vi "Meas_EIS_Spectra_Polar_v6.vi"(9 "output cluster":T1, 10 "testp":T2={"Start F"=1.0, "Stop F"=10000.0, "# Steps"=50, "Init Z Guess"=1.0, "Device #"=0, "Vdrive (V)"=0.1} caption="Test Parameters" {"Vdrive (V)" min=0.0001 max=10; "Device #" min=0 max=10 step=1; "Init Z Guess" format="%_5f"; "# Steps" min=1 max=1800 step=1; "Stop F" min=0.0010000000474974513 max=2000000.0 step=0.001 format="%#_3f"; "Start F" min=0.0010000000474974513 max=2000000.0 step=0.001 format="%#_3f"}, 11 "Output file refnum":refnum<file>) -> ()   [LabVIEW 2018]
uses:
  AC States cntrl.ctl
panel:
  out "Init Z Guess":sgl
  in  "Tab Control":enum32{"Outputs", "TakeData"}(tab)
  out "XY Graph":cluster{sgl, sgl}[](graph)
  out "IERange":i32
  out "IchRange":i32
  out "VchRange":i32
  out "Index no.":i32=1
  out "Zphz":dbl
  out "Zmod":dbl
  out "Zfreq":dbl
  in  "Control Mode":i32(ring)=1 items=["GstatMode", "PstatMode", "ZRAMode", "FRAMode"]
  out "Data Available":bool
  out "Status":enum16{"Ok", "Retry", "Error", "Done"}(ring)
  out "NumPoints":i32
  in  "Freqin":sgl=1000.0 format="%#_3g"
  out "event callback refnum":refnum<k27>
  out "Section":string
  out "ReadZ":refnum<k7>
  out "Pstat":refnum<k7>
  out "Device List":refnum<k7>
  out "Data Acquisition Complete":bool
  in  "GAMRYCOMLib.IGamryReadZ":refnum<k7>
  in  "GAMRYCOMLib.IGamryPstat":refnum<k7>
  in  "GAMRYCOMLib.IGamryDeviceList":refnum<k7>
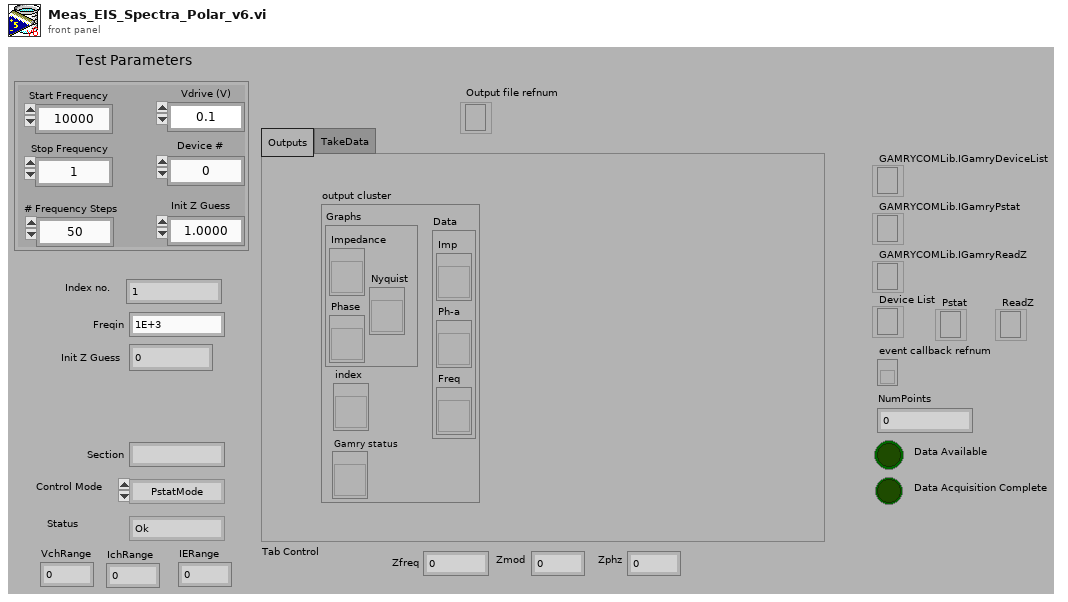
[diagram p1: front panel]
types:
  T1 = cluster{"Data":cluster{"Imp":refnum<vi>, "Ph-a":refnum<vi>, "Freq":refnum<vi>}, "Graphs":cluster{"Impedance":refnum<vi>, "Phase":refnum<vi>, "Nyquist":refnum<vi>}, "index":refnum<vi>, "Gamry status":refnum<vi>}
  T2 = cluster{"Start F":dbl, "Stop F":dbl, "# Steps":u32, "Init Z Guess":sgl, "Device #":i16, "Vdrive (V)":sgl}
  T3 = typedef "AC States cntrl.ctl" = enum16{"Initialize Variables", "Initialize Pstat", "Initialize Dtaq", "Settings", "Frequency calc", "Set Cycle Limits", "Take Data", "Read Z Measure", "Cleanup", "Stop"}
  T4 = cluster{"Imp":refnum<vi>, "Ph-a":refnum<vi>, "Freq":refnum<vi>}
  T5 = cluster{"Impedance":refnum<vi>, "Phase":refnum<vi>, "Nyquist":refnum<vi>}
  T6 = cluster{"Data Acquisition Complete":refnum<vi>, "Status":refnum<vi>}
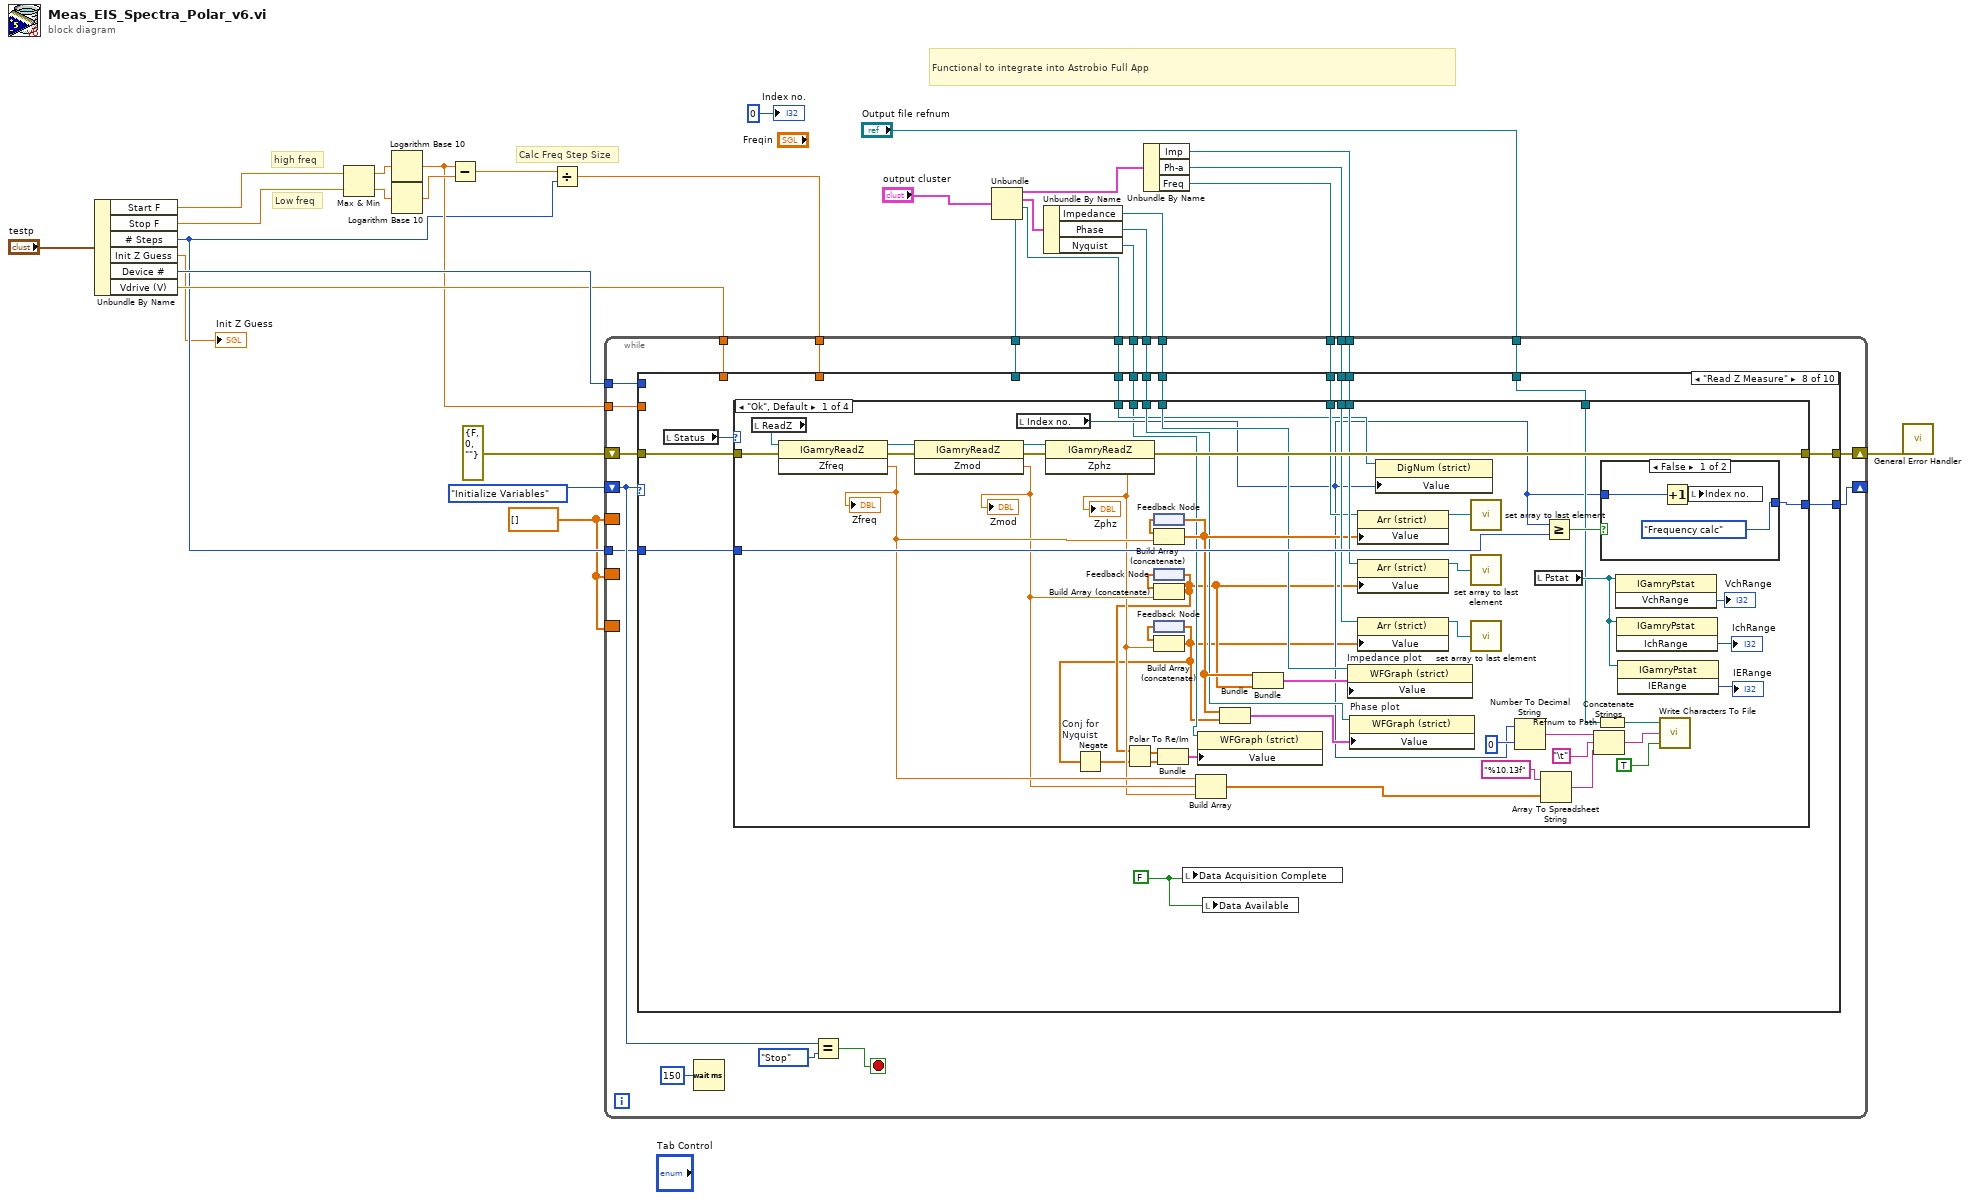
[diagram p0: block diagram]
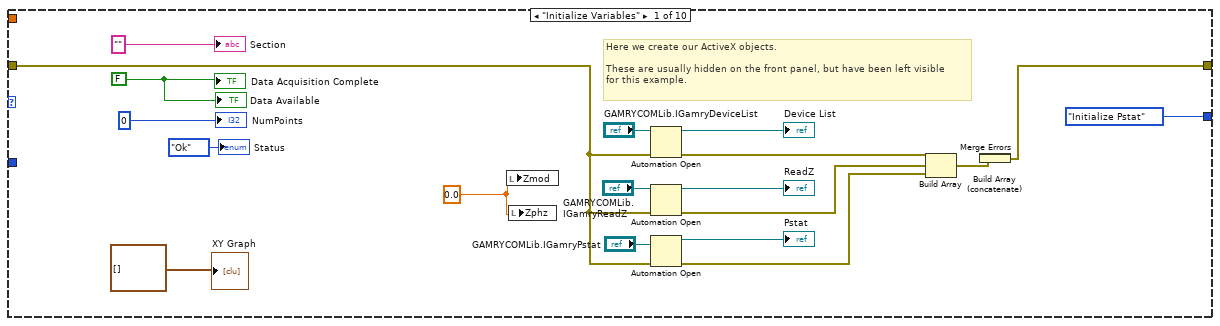
[diagram p2: hidden frame]
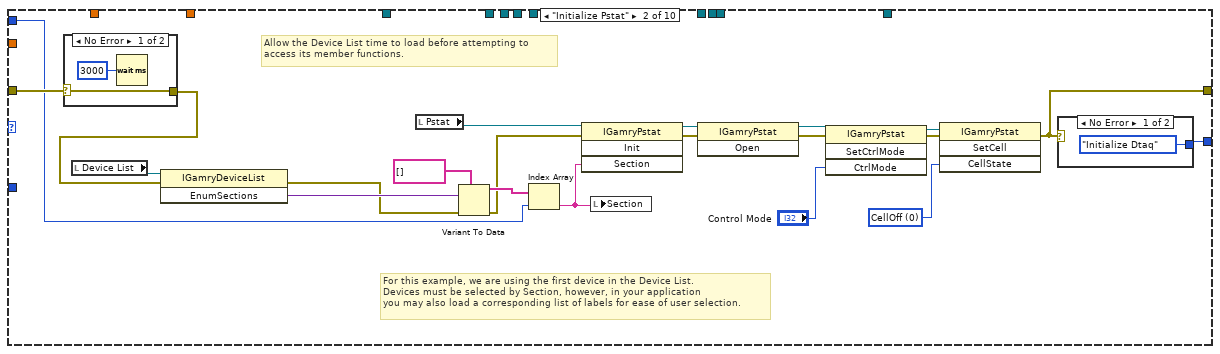
[diagram p3: hidden frame]
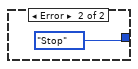
[diagram p5: hidden frame]
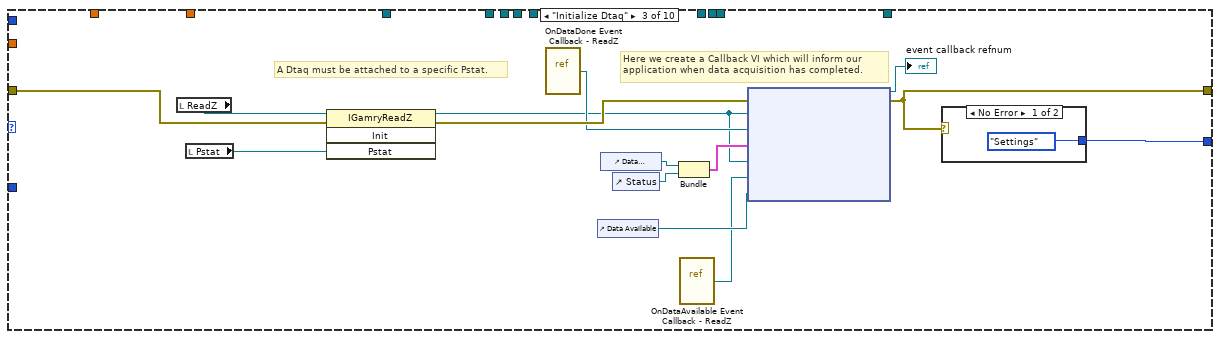
[diagram p6: hidden frame]
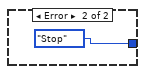
[diagram p7: hidden frame]
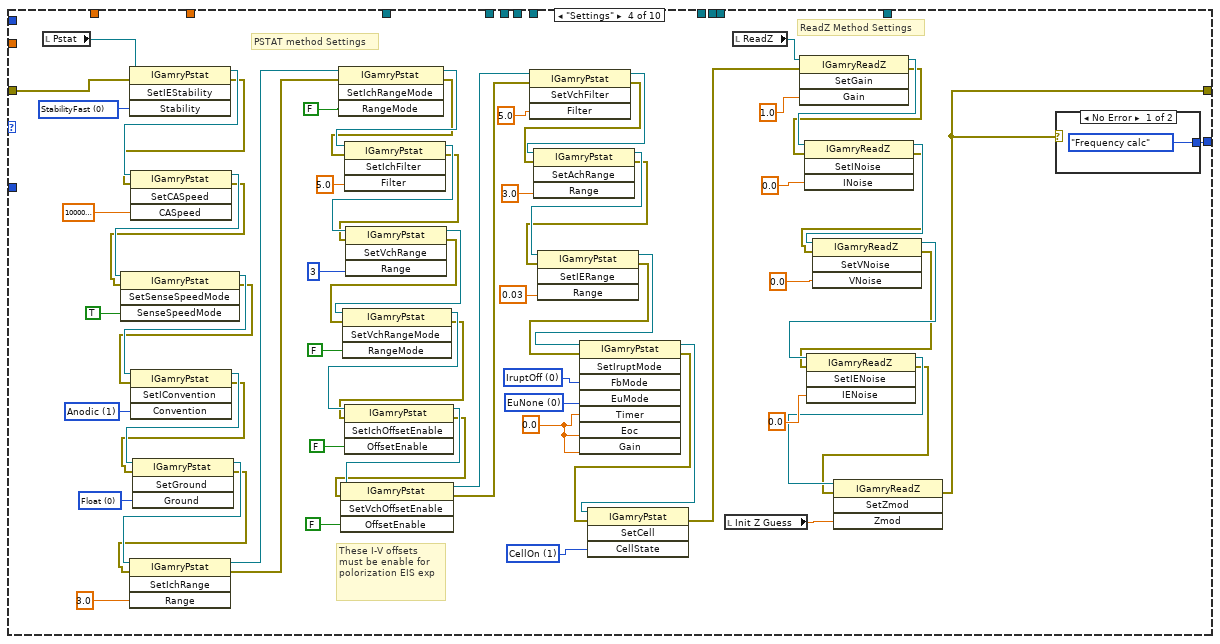
[diagram p8: hidden frame]
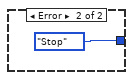
[diagram p9: hidden frame]
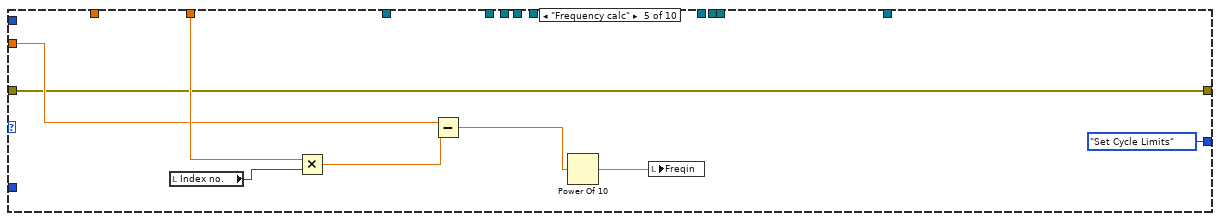
[diagram p10: hidden frame]
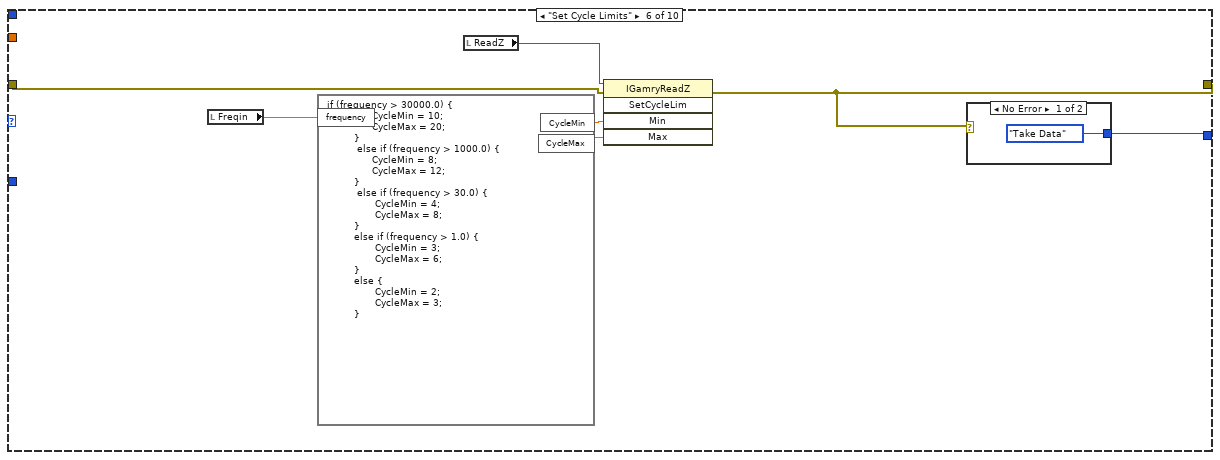
[diagram p11: hidden frame]
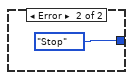
[diagram p12: hidden frame]
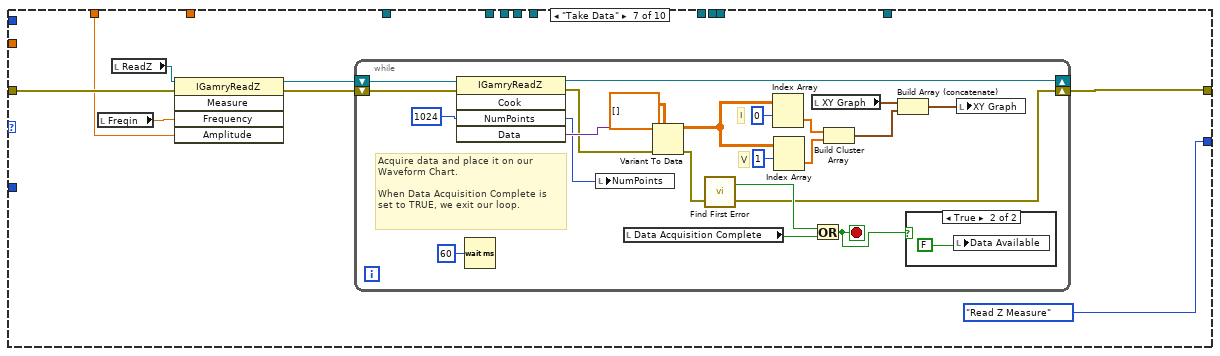
[diagram p13: hidden frame]
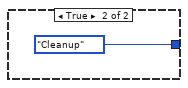
[diagram p15: hidden frame]
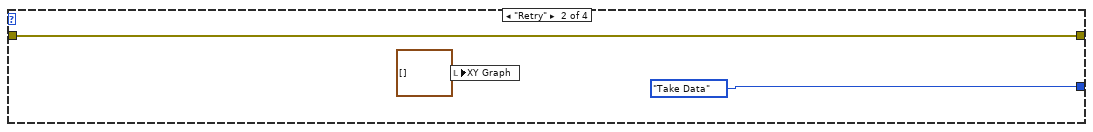
[diagram p16: hidden frame]
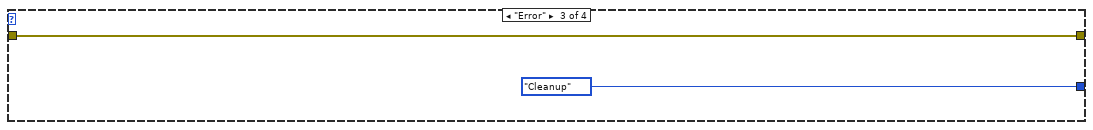
[diagram p17: hidden frame]
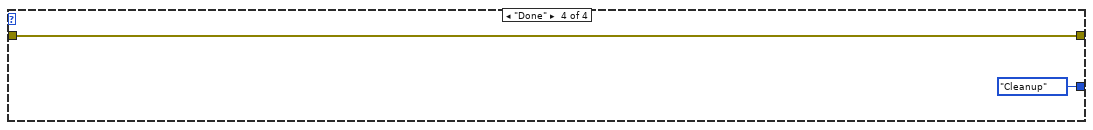
[diagram p18: hidden frame]
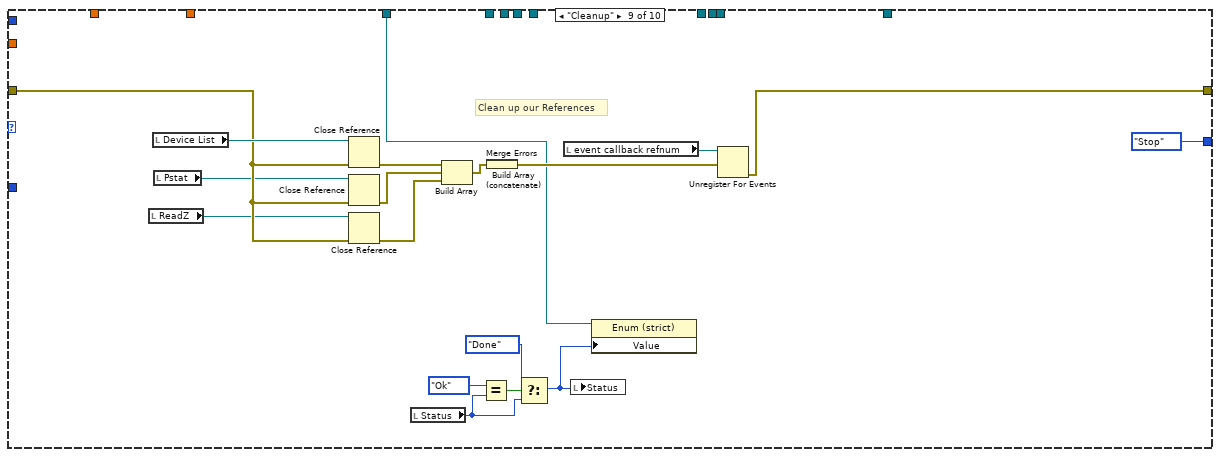
[diagram p19: hidden frame]
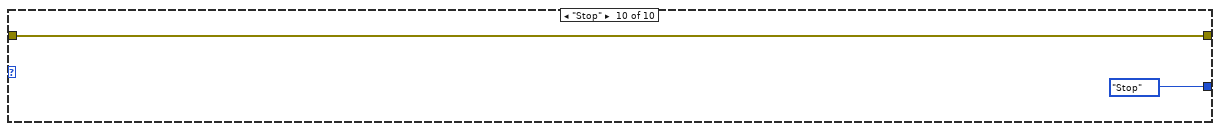
[diagram p20: hidden frame]
diagram:
  w4 = dbl[] []
  # "Functional to integrate into Astrobio Full App"
  # "Calc Freq Step Size"
  # "Low freq"
  # "high freq"
  n1 = Unbundle By Name("testp") -> ("Start F"=w20:dbl, "Stop F"=w19:dbl, "# Steps"=w15:u32, "Init Z Guess"=→"Init Z Guess":sgl, "Device #"=w26:i16, "Vdrive (V)"=w25:sgl)
  n2 = Max & Min(x=w20, y=w19) -> (max(x,y)=w23:dbl, min(x,y)=w24:dbl)
  n3 = Logarithm Base 10(1:w23) -> (0:w17:dbl)
  n4 = Logarithm Base 10(1:w24) -> (0:w21:dbl)
  n5 = Subtract(x=w17, y=w21) -> (x-y=w22:dbl)
  n6 = Divide(x=w22, y=w15) -> (x/y=w16:dbl)
  n7 = Unbundle("output cluster") -> ("Data"=w11:T4, "Graphs"=w7:T5, "index"=w2:refnum<vi>, "Gamry status"=w3:refnum<vi>)
  n8 = Unbundle By Name(w7) -> ("Impedance"=w6:refnum<vi>, "Phase"=w5:refnum<vi>, "Nyquist"=w1:refnum<vi>)
  n9 = Unbundle By Name(w11) -> ("Imp"=w10:refnum<vi>, "Ph-a"=w9:refnum<vi>, "Freq"=w8:refnum<vi>)
  n10 = while {
    shift-right: [w48] -> _
    shift-left: AC_States_cntrl."Initialize Variables" ("DC Demo States") -> [w49]
    shift-right: [w46] -> w29
    shift-left: errorcluster {"status"=FALSE, "code"=0, "source"=""} ("error in (no error)") -> [w47]
    tunnel: w25 -> [w44]
    tunnel: w26 -> [w43]
    tunnel: w15 -> [w42]
    tunnel: w17 -> [w41]
    tunnel: w16 -> [w40]
    tunnel: "Output file refnum" -> [w39]
    border: w4 -> [_]
    border: w4 -> [_]
    border: w4 -> [_]
    tunnel: w10 -> [w38]
    tunnel: w9 -> [w37]
    tunnel: w8 -> [w36]
    tunnel: w6 -> [w35]
    tunnel: w5 -> [w34]
    tunnel: w2 -> [w33]
    tunnel: w3 -> [w32]
    tunnel: w1 -> [w31]
    stop <- w50 stop-if-true
    n11 = case shown="\"Read Z Measure\"" w49 {
      tunnel: [AC_States_cntrl."Initialize Pstat" ("DC Demo States") w88 w110 w182 AC_States_cntrl."Set Cycle Limits" ("DC Demo States") w200 AC_States_cntrl."Read Z Measure" ("DC Demo States") w246 AC_States_cntrl."Stop" ("DC Demo States") AC_States_cntrl."Stop" ("DC Demo States")] -> w48
      tunnel: w47 -> [w60 w79 w108 w163 w186 w199 w209 w245 w325 w328]
      tunnel: [w61 w72 w107 w181 w186 w194 w208 w244 w316 w328] -> w46
      tunnel: w44 -> [_ _ _ _ _ _ w204 _ _ _]
      tunnel: w43 -> [_ w76 _ _ _ _ _ _ _ _]
      tunnel: w42 -> [_ _ _ _ _ _ _ w243 _ _]
      tunnel: w41 -> [_ _ _ _ w191 _ _ _ _ _]
      tunnel: w40 -> [_ _ _ _ w192 _ _ _ _ _]
      tunnel: w39 -> [_ _ _ _ _ _ _ w242 _ _]
      tunnel: w38 -> [_ _ _ _ _ _ _ w240 _ _]
      tunnel: w37 -> [_ _ _ _ _ _ _ w239 _ _]
      tunnel: w36 -> [_ _ _ _ _ _ _ w238 _ _]
      tunnel: w35 -> [_ _ _ _ _ _ _ w237 _ _]
      tunnel: w34 -> [_ _ _ _ _ _ _ w236 _ _]
      tunnel: w33 -> [_ _ _ _ _ _ _ w235 _ _]
      tunnel: w32 -> [_ _ _ _ _ _ _ _ w313 _]
      tunnel: w31 -> [_ _ _ _ _ _ _ w234 _ _]
      frame "Initialize Variables" {
        w54 = sgl 0.0 ("Zreal")
        w56 = FALSE
        # "Here we create our ActiveX objects.\n\nThese are usually hidden on the front panel, but have been left visible\nfor this example."
        n12 = local write "Zmod"(w54) -> ()
        n13 = local write "Zphz"(w54) -> ()
        n14 = Automation Open(error in (no error)=w60, Automation Refnum="GAMRYCOMLib.IGamryDeviceList") -> (Automation Refnum=→"Device List":refnum<k7>, error out=w63:errorcluster)  [unwired: 2 in]
        n15 = Automation Open(error in (no error)=w60, Automation Refnum="GAMRYCOMLib.IGamryReadZ") -> (Automation Refnum=→"ReadZ":refnum<k7>, error out=w58:errorcluster)  [unwired: 2 in]
        n16 = Automation Open(error in (no error)=w60, Automation Refnum="GAMRYCOMLib.IGamryPstat") -> (Automation Refnum=→"Pstat":refnum<k7>, error out=w59:errorcluster)  [unwired: 2 in]
        n17 = Build Array(w63, w58, w59) -> (w62:errorcluster[])
        n18 = Build Array (concatenate)(w62) -> (w55:errorcluster[])
        n19 = Merge Errors(w55) -> (w61:errorcluster)
        "Data Acquisition Complete" <- w56
        "Section" <- "" ("Section")
        "NumPoints" <- 0 ("NumPoints")
        "Data Available" <- w56
        "XY Graph" <- cluster{sgl, sgl}[] [] ("appended array")
        "Status" <- enum16{"Ok", "Retry", "Error", "Done"}."Ok" ("Status")
      }
      frame "Initialize Pstat" {
        w75 = 0 items=["CellOff", "CellOn"] ("CellState")
        # "For this example, we are using the first device in the Device List.\nDevices must be selected by Section, however, in your application\nyou may also load a corresponding list of labels for ease of user selection."
        # "Allow the Device List time to load before attempting to \naccess its member functions."
        n20 = case shown="No Error" w79 {
          selector: w79 -> [w93 w95]
          tunnel: [w93 w95] -> w78
          frame No Error {
            n21 = Wait (ms)(milliseconds to wait=u32 3000) -> ()  [unwired: 1 out]
          }
          frame Error {
          }
        }
        n22 = local read "Device List"() -> (w83:refnum<k7>)
        n23 = invoke class="IGamryDeviceList" method="EnumSections"(reference=w83, error in=w78) -> (error out=w81:errorcluster, "EnumSections"=w82:variant)  [unwired: 1 in, 1 out]
        n24 = local read "Pstat"() -> (w85:refnum<k7>)
        n25 = Variant To Data(error in=w81, type=string[] [], Variant=w82) -> (data=w87:string[], error out=w80:errorcluster)
        n26 = Index Array(array=w87, index=w76) -> (element=w84:string)
        n27 = invoke class="IGamryPstat" method="Init"(reference=w85, error in=w80, "Section"=w84) -> (reference out=w92:refnum<k7>, error out=w91:errorcluster)  [unwired: 1 in, 2 out]
        n28 = local write "Section"(w84) -> ()
        n29 = invoke class="IGamryPstat" method="Open"(reference=w92, error in=w91) -> (reference out=w89:refnum<k7>, error out=w90:errorcluster)  [unwired: 1 in, 1 out]
        n30 = invoke class="IGamryPstat" method="SetCtrlMode"(reference=w89, error in=w90, "CtrlMode"="Control Mode") -> (reference out=w74:refnum<k7>, error out=w73:errorcluster)  [unwired: 1 in, 2 out]
        n31 = invoke class="IGamryPstat" method="SetCell"(reference=w74, error in=w73, "CellState"=w75) -> (error out=w72:errorcluster)  [unwired: 1 in, 3 out]
        n32 = case shown="No Error" w72 {
          tunnel: [AC_States_cntrl."Initialize Dtaq" ("DC Demo States") AC_States_cntrl."Stop" ("DC Demo States")] -> w88
          frame No Error {
          }
          frame Error {
          }
        }
      }
      frame "Initialize Dtaq" {
        # "A Dtaq must be attached to a specific Pstat."
        # "Here we create a Callback VI which will inform our\napplication when data acquisition has completed."
        n33 = local read "ReadZ"() -> (w109:refnum<k7>)
        n34 = local read "Pstat"() -> (w111:refnum<k7>)
        n35 = invoke class="IGamryReadZ" method="Init"(reference=w109, error in=w108, "Pstat"=w111) -> (reference out=w99:refnum<k7>, error out=w105:errorcluster)  [unwired: 1 in, 2 out]
        n36 = vi-ref "OnDataDone Event Callback - ReadZ.vi"() -> ("vi reference"=w101:refnum<vi>)
        n37 = control-ref of="Data Available"() -> (w100:refnum<vi>)
        n38 = control-ref of="Data Acquisition Complete"() -> (w104:refnum<vi>)
        n39 = control-ref of="Status"() -> (w103:refnum<vi>)
        n40 = Bundle("Data Acquisition Complete"=w104, "Status"=w103) -> (w102:T6)  [unwired: 1 in]
        n41 = vi-ref "OnDataAvailable Event Callback - ReadZ.vi"() -> ("vi reference"=w98:refnum<vi>)
        n42 = node(w105, w99, w101, w102, w99, w98, w100) -> (→"event callback refnum":refnum<k27>, w107:errorcluster)  [unwired: 1 in]
        n43 = case shown="No Error" w107 {
          tunnel: [AC_States_cntrl."Settings" ("DC Demo States") AC_States_cntrl."Stop" ("DC Demo States")] -> w110
          frame No Error {
          }
          frame Error {
          }
        }
      }
      frame "Settings" {
        w117 = sgl 0.0 ("Timer")
        w118 = 0 items=["EuNone", "EuExtrap", "EuAverage"] ("EuMode")
        w119 = 0 items=["IruptOff", "IruptNorm", "IruptClfg"] ("FbMode")
        w152 = 0 items=["Float", "Earth"] ("Ground")
        w155 = 1 items=["Cathodic", "Anodic"] ("Convention")
        w162 = 0 items=["StabilityFast", "StabilityMedFast", "StabilityNorm", "StabilitySlow"] ("Stability")
        w183 = 1 items=["CellOff", "CellOn"] ("CellState")
        # "ReadZ Method Settings"
        # "These I-V offsets must be enable for polorization EIS exp"
        # "PSTAT method Settings"
        n44 = local read "Pstat"() -> (w164:refnum<k7>)
        n45 = invoke class="IGamryPstat" method="SetIEStability"(reference=w164, error in=w163, "Stability"=w162) -> (reference out=w161:refnum<k7>, error out=w160:errorcluster)  [unwired: 1 in, 2 out]
        n46 = invoke class="IGamryPstat" method="SetCASpeed"(reference=w161, error in=w160, "CASpeed"=1000000.0) -> (reference out=w157:refnum<k7>, error out=w156:errorcluster)  [unwired: 1 in, 2 out]
        n47 = invoke class="IGamryPstat" method="SetSenseSpeedMode"(reference=w157, error in=w156, "SenseSpeedMode"=TRUE) -> (reference out=w154:refnum<k7>, error out=w153:errorcluster)  [unwired: 1 in, 2 out]
        n48 = invoke class="IGamryPstat" method="SetIConvention"(reference=w154, error in=w153, "Convention"=w155) -> (reference out=w151:refnum<k7>, error out=w150:errorcluster)  [unwired: 1 in, 2 out]
        n49 = invoke class="IGamryPstat" method="SetGround"(reference=w151, error in=w150, "Ground"=w152) -> (reference out=w148:refnum<k7>, error out=w147:errorcluster)  [unwired: 1 in, 2 out]
        n50 = invoke class="IGamryPstat" method="SetIchRange"(reference=w148, error in=w147, "Range"=3.0) -> (reference out=w146:refnum<k7>, error out=w145:errorcluster)  [unwired: 1 in, 2 out]
        n51 = invoke class="IGamryPstat" method="SetIchRangeMode"(reference=w146, error in=w145, "RangeMode"=FALSE) -> (reference out=w142:refnum<k7>, error out=w141:errorcluster)  [unwired: 1 in, 2 out]
        n52 = invoke class="IGamryPstat" method="SetIchFilter"(reference=w142, error in=w141, "Filter"=5.0) -> (reference out=w140:refnum<k7>, error out=w139:errorcluster)  [unwired: 1 in, 2 out]
        n53 = invoke class="IGamryPstat" method="SetVchRange"(reference=w140, error in=w139, "Range"=3) -> (reference out=w137:refnum<k7>, error out=w136:errorcluster)  [unwired: 1 in, 2 out]
        n54 = invoke class="IGamryPstat" method="SetVchRangeMode"(reference=w137, error in=w136, "RangeMode"=FALSE) -> (reference out=w135:refnum<k7>, error out=w134:errorcluster)  [unwired: 1 in, 2 out]
        n55 = invoke class="IGamryPstat" method="SetIchOffsetEnable"(reference=w135, error in=w134, "OffsetEnable"=FALSE) -> (reference out=w131:refnum<k7>, error out=w130:errorcluster)  [unwired: 1 in, 2 out]
        n56 = invoke class="IGamryPstat" method="SetVchOffsetEnable"(reference=w131, error in=w130, "OffsetEnable"=FALSE) -> (reference out=w129:refnum<k7>, error out=w128:errorcluster)  [unwired: 1 in, 2 out]
        n57 = invoke class="IGamryPstat" method="SetVchFilter"(reference=w129, error in=w128, "Filter"=5.0) -> (reference out=w125:refnum<k7>, error out=w124:errorcluster)  [unwired: 1 in, 2 out]
        n58 = invoke class="IGamryPstat" method="SetAchRange"(reference=w125, error in=w124, "Range"=3.0) -> (reference out=w123:refnum<k7>, error out=w122:errorcluster)  [unwired: 1 in, 2 out]
        n59 = invoke class="IGamryPstat" method="SetIERange"(reference=w123, error in=w122, "Range"=0.03) -> (reference out=w121:refnum<k7>, error out=w120:errorcluster)  [unwired: 1 in, 2 out]
        n60 = invoke class="IGamryPstat" method="SetIruptMode"(reference=w121, error in=w120, "FbMode"=w119, "EuMode"=w118, "Timer"=w117, "Eoc"=w117, "Gain"=w117) -> (reference out=w116:refnum<k7>, error out=w115:errorcluster)  [unwired: 1 in, 6 out]
        n61 = invoke class="IGamryPstat" method="SetCell"(reference=w116, error in=w115, "CellState"=w183) -> (error out=w178:errorcluster)  [unwired: 1 in, 3 out]
        n62 = local read "Init Z Guess"() -> (w114:sgl)
        n63 = local read "ReadZ"() -> (w179:refnum<k7>)
        n64 = invoke class="IGamryReadZ" method="SetGain"(reference=w179, error in=w178, "Gain"=sgl 1.0 ("Zmod")) -> (reference out=w176:refnum<k7>, error out=w175:errorcluster)  [unwired: 1 in, 2 out]
        n65 = invoke class="IGamryReadZ" method="SetINoise"(reference=w176, error in=w175, "INoise"=sgl 0.0 ("Zmod")) -> (reference out=w173:refnum<k7>, error out=w172:errorcluster)  [unwired: 1 in, 2 out]
        n66 = invoke class="IGamryReadZ" method="SetVNoise"(reference=w173, error in=w172, "VNoise"=sgl 0.0 ("Zmod")) -> (reference out=w170:refnum<k7>, error out=w169:errorcluster)  [unwired: 1 in, 2 out]
        n67 = invoke class="IGamryReadZ" method="SetIENoise"(reference=w170, error in=w169, "IENoise"=sgl 0.0 ("Zmod")) -> (reference out=w168:refnum<k7>, error out=w167:errorcluster)  [unwired: 1 in, 2 out]
        n68 = invoke class="IGamryReadZ" method="SetZmod"(reference=w168, error in=w167, "Zmod"=w114) -> (error out=w181:errorcluster)  [unwired: 1 in, 3 out]
        n69 = case shown="No Error" w181 {
          tunnel: [AC_States_cntrl."Frequency calc" ("DC Demo States") AC_States_cntrl."Stop" ("DC Demo States")] -> w182
          frame No Error {
          }
          frame Error {
          }
        }
      }
      frame "Frequency calc" {
        n70 = local read "Index no."() -> (w193:i32)
        n71 = Multiply(x=w192, y=w193) -> (x*y=w190:dbl)
        n72 = Subtract(x=w191, y=w190) -> (x-y=w189:dbl)
        n73 = Power Of 10(x=w189) -> (10^x=w188:dbl)
        n74 = local write "Freqin"(w188) -> ()
      }
      frame "Set Cycle Limits" {
        n75 = local read "Freqin"() -> (w197:sgl)
        n76 = formula code="if (frequency > 30000.0) {\n               CycleMin = 10;\n               CycleMax = 20;\n         }\n          else if (frequency > 1000.0) {\n               CycleMin = 8;\n               CycleMax = 12;\n         }\n          else if (frequency > 30.0) {\n                CycleMin = 4;\n                CycleMax = 8;\n         }\n         else if (frequency > 1.0) {\n                CycleMin = 3;\n                CycleMax = 6;\n         }\n         else {\n                CycleMin = 2;\n                CycleMax = 3;\n         }"("frequency"=w197) -> ("CycleMin"=w196:dbl, "CycleMax"=w195:dbl)
        n77 = local read "ReadZ"() -> (w198:refnum<k7>)
        n78 = invoke class="IGamryReadZ" method="SetCycleLim"(reference=w198, error in=w199, "Min"=w196, "Max"=w195) -> (error out=w194:errorcluster)  [unwired: 1 in, 4 out]
        n79 = case shown="No Error" w194 {
          tunnel: [AC_States_cntrl."Take Data" ("DC Demo States") AC_States_cntrl."Stop" ("DC Demo States")] -> w200
          frame No Error {
          }
          frame Error {
          }
        }
      }
      frame "Take Data" {
        n80 = local read "Freqin"() -> (w203:sgl)
        n81 = local read "ReadZ"() -> (w207:refnum<k7>)
        n82 = invoke class="IGamryReadZ" method="Measure"(reference=w207, error in=w209, "Frequency"=w203, "Amplitude"=w204) -> (reference out=w206:refnum<k7>, error out=w205:errorcluster)  [unwired: 1 in, 3 out]
        n83 = while {
          shift-right: [w223] -> w208
          shift-left: w205 -> [w231]
          shift-right: [w222] -> _
          shift-left: w206 -> [w232]
          stop <- w211 stop-if-true
          # "V"
          # "I"
          # "Acquire data and place it on our\nWaveform Chart.\n\nWhen Data Acquisition Complete is\nset to TRUE, we exit our loop."
          n84 = invoke class="IGamryReadZ" method="Cook"(reference=w232, error in=w231, "NumPoints"=1024) -> (reference out=w222:refnum<k7>, error out=w227:errorcluster, "NumPoints"=w217:i32, "Data"=w228:variant)  [unwired: 2 in, 1 out]
          n85 = Wait (ms)(milliseconds to wait=u32 60) -> ()  [unwired: 1 out]
          n86 = local write "NumPoints"(w217) -> ()
          n87 = local read "Data Acquisition Complete"() -> (w224:bool)
          n88 = Variant To Data(error in=w227, type=sgl[][] [], Variant=w228) -> (data=w218:sgl[][], error out=w226:errorcluster)
          n89 = call <vilib>:"Find First Error.vi"("error in (no error)"=w226) -> ("error out"=w223:errorcluster, "error?"=w225:bool)  [unwired: 3 in]
          n90 = Index Array(array=w218, index (row)=0) -> (element=w216:sgl[])  [unwired: 1 in]
          n91 = Index Array(array=w218, index (row)=1) -> (element=w215:sgl[])  [unwired: 1 in]
          n92 = local read "XY Graph"() -> (w214:cluster{sgl, sgl}[])
          n93 = Or(x=w225, y=w224) -> (x .or. y?=w211:bool)
          n94 = Build Cluster Array(w216, w215) -> (w213:cluster{sgl, sgl}[])
          n95 = Build Array (concatenate)(w214, w213) -> (w212:cluster{sgl, sgl}[])
          n96 = case shown="True" w211 {
            frame False {
            }
            frame True {
              n97 = local write "Data Available"(FALSE) -> ()
            }
          }
          n98 = local write "XY Graph"(w212) -> ()
        }
      }
      frame "Read Z Measure" {
        w241 = FALSE
        n99 = local read "Status"() -> (w247:enum16{"Ok", "Retry", "Error", "Done"})
        n100 = case shown="\"Ok\", Default" w247 {
          tunnel: [w284 AC_States_cntrl."Take Data" ("DC Demo States") AC_States_cntrl."Cleanup" ("DC Demo States") AC_States_cntrl."Cleanup" ("DC Demo States")] -> w246
          tunnel: w245 -> [w294 w303 w305 w308]
          tunnel: [w295 w303 w305 w308] -> w244
          tunnel: w243 -> [w286 _ _ _]
          tunnel: w242 -> [w275 _ _ _]
          tunnel: w240 -> [w267 _ _ _]
          tunnel: w239 -> [w266 _ _ _]
          tunnel: w238 -> [w265 _ _ _]
          tunnel: w237 -> [w261 _ _ _]
          tunnel: w236 -> [w260 _ _ _]
          tunnel: w235 -> [w259 _ _ _]
          tunnel: w234 -> [w253 _ _ _]
          frame "Ok", Default {
            n101 = local read "ReadZ"() -> (w291:refnum<k7>)
            n102 = invoke class="IGamryReadZ" method="Zfreq"(reference=w291, error in=w294) -> (reference out=w292:refnum<k7>, error out=w293:errorcluster, "Zfreq"=w271:sgl)  [unwired: 1 in]
            "Zfreq" <- w271
            n103 = invoke class="IGamryReadZ" method="Zmod"(reference=w292, error in=w293) -> (reference out=w296:refnum<k7>, error out=w297:errorcluster, "Zmod"=w270:sgl)  [unwired: 1 in]
            "Zmod" <- w270
            n104 = local read "Index no."() -> (w258:i32)
            n105 = invoke class="IGamryReadZ" method="Zphz"(reference=w296, error in=w297) -> (error out=w295:errorcluster, "Zphz"=w268:sgl)  [unwired: 1 in, 1 out]
            "Zphz" <- w268
            n106 = feedback #1() -> (w256:dbl[])
            n107 = Build Array (concatenate)(w256, w271) -> (w263:dbl[])
            n108 = feedback-in #1(w263) -> ()
            n109 = feedback #2() -> (w269:dbl[])
            n110 = Build Array (concatenate)(w269, w270) -> (w250:dbl[])
            n111 = feedback-in #2(w250) -> ()
            n112 = feedback #3() -> (w257:dbl[])
            n113 = Build Array (concatenate)(w257, w268) -> (w249:dbl[])
            n114 = Negate "Conj for\nNyquist"(x=w249) -> (-x=w248:dbl[])
            n115 = Polar To Re/Im(2:w248, 3:w250) -> (0:w251:dbl[], 1:w252:dbl[])
            n116 = feedback-in #3(w249) -> ()
            n117 = Bundle(w252, w251) -> (w254:cluster{dbl[], dbl[]})  [unwired: 1 in]
            n118 = Build Array(w271, w270, w268) -> (w281:sgl[])
            n119 = property class="WFGraph (strict)"(reference=w253, "Value"=w254) -> ()  [unwired: 1 in, 2 out]
            n120 = Bundle(w263, w249) -> (w262:cluster{dbl[], dbl[]})  [unwired: 1 in]
            n121 = Bundle(w263, w250) -> (w264:cluster{dbl[], dbl[]})  [unwired: 1 in]
            n122 = property on="Impedance plot" class="WFGraph (strict)"(reference=w261, "Value"=w264) -> ()  [unwired: 1 in, 2 out]
            n123 = property on="Phase plot" class="WFGraph (strict)"(reference=w260, "Value"=w262) -> ()  [unwired: 1 in, 2 out]
            n124 = property class="Arr (strict)"(reference=w265, "Value"=w263) -> (reference out=w274:refnum<vi>)  [unwired: 1 in, 1 out]
            n125 = property class="Arr (strict)"(reference=w267, "Value"=w250) -> (reference out=w273:refnum<vi>)  [unwired: 1 in, 1 out]
            n126 = property class="Arr (strict)"(reference=w266, "Value"=w249) -> (reference out=w272:refnum<vi>)  [unwired: 1 in, 1 out]
            n127 = property class="DigNum (strict)"(reference=w259, "Value"=w258) -> ()  [unwired: 1 in, 2 out]
            n128 = call "set array to last element.vi"("Arr Refnum"=w274) -> ()
            n129 = call "set array to last element.vi"("Arr Refnum"=w273) -> ()
            n130 = call "set array to last element.vi"("Arr Refnum"=w272) -> ()
            n131 = Number To Decimal String(number=w258, width (-)=i16 0) -> (decimal integer string=w278:string)
            n132 = local read "Pstat"() -> (w290:refnum<k7>)
            n133 = Array To Spreadsheet String(array=w281, 3:"%10.13f") -> (spreadsheet string=w277:string)  [unwired: 1 in]
            n134 = Greater Or Equal?(x=w258, y=w286) -> (x >= y?=w285:bool)
            n135 = Concatenate Strings(w278, "\t", w277) -> (w276:string)
            n136 = Refnum to Path(1:w275) -> (0:w255:path)
            n137 = case shown="False" w285 {
              tunnel: [AC_States_cntrl."Frequency calc" ("DC Demo States") AC_States_cntrl."Cleanup" ("DC Demo States")] -> w284
              tunnel: w258 -> [w298 _]
              frame False {
                n138 = Increment(x=w298) -> (x+1=w299:i32)
                n139 = local write "Index no."(w299) -> ()
              }
              frame True {
              }
            }
            n140 = invoke class="IGamryPstat" method="VchRange"(reference=w290) -> ("VchRange"=→"VchRange":i32)  [unwired: 2 in, 2 out]
            n141 = invoke class="IGamryPstat" method="IchRange"(reference=w290) -> ("IchRange"=→"IchRange":i32)  [unwired: 2 in, 2 out]
            n142 = invoke class="IGamryPstat" method="IERange"(reference=w290) -> ("IERange"=→"IERange":i32)  [unwired: 2 in, 2 out]
            n143 = call <vilib>:"Write Characters To File.vi"("append to file? (new file:F)"=TRUE, "character string"=w276, "file path (dialog if empty)"=w255) -> ()  [unwired: 2 in, 1 out]
          }
          frame "Retry" {
            n144 = local write "XY Graph"(cluster{sgl, sgl}[] [] ("appended array")) -> ()
          }
          frame "Error" {
          }
          frame "Done" {
          }
        }
        n145 = local write "Data Acquisition Complete"(w241) -> ()
        n146 = local write "Data Available"(w241) -> ()
      }
      frame "Cleanup" {
        # "Clean up our References"
        n147 = local read "ReadZ"() -> (w323:refnum<k7>)
        n148 = local read "Device List"() -> (w326:refnum<k7>)
        n149 = local read "Pstat"() -> (w324:refnum<k7>)
        n150 = Close Reference(reference=w326, error in (no error)=w325) -> (error out=w322:errorcluster)
        n151 = Close Reference(reference=w324, error in (no error)=w325) -> (error out=w321:errorcluster)
        n152 = Close Reference(reference=w323, error in (no error)=w325) -> (error out=w320:errorcluster)
        n153 = local read "Status"() -> (w309:enum16{"Ok", "Retry", "Error", "Done"})
        n154 = Build Array(w322, w321, w320) -> (w319:errorcluster[])
        n155 = Equal?(x=enum16{"Ok", "Retry", "Error", "Done"}."Ok", y=w309) -> (x = y?=w314:bool)
        n156 = Build Array (concatenate)(w319) -> (w315:errorcluster[])
        n157 = Merge Errors(w315) -> (w317:errorcluster)
        n158 = Select(t=enum16{"Ok", "Retry", "Error", "Done"}."Done", s=w314, f=w309) -> (s? t:f=w312:enum16{"Ok", "Retry", "Error", "Done"})
        n159 = local read "event callback refnum"() -> (w318:refnum<k27>)
        n160 = local write "Status"(w312) -> ()
        n161 = property class="Enum (strict)"(reference=w313, "Value"=w312) -> ()  [unwired: 1 in, 2 out]
        n162 = Unregister For Events(event registration refnum=w318, error in=w317) -> (error out=w316:errorcluster)
      }
      frame "Stop" {
      }
    }
    n163 = Wait (ms)(milliseconds to wait=u32 150) -> ()  [unwired: 1 out]
    n164 = Equal?(x=w49, y=AC_States_cntrl."Stop" ("DC Demo States")) -> (x = y?=w50:bool)
  }
  n165 = call <vilib>:"General Error Handler.vi"("error in (no error)"=w29) -> ()  [unwired: 10 in, 5 out]
  "Index no." <- 0 ("Index no.")
